vi "GetTaskTypeByTaskID.vi"(3 "Task ID":u32) -> (0 "task type":i32, 1 "Task ID":u32)   [LabVIEW 2009]
uses:
  Windows/System32/AdvLvDaq.dll
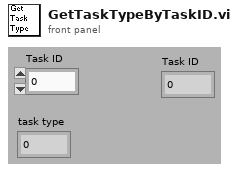
[diagram p1: front panel]
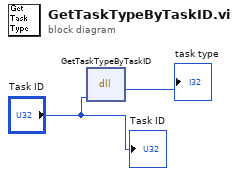
[diagram p0: block diagram]
diagram:
  n1 = dll-call lib="C:/Windows/System32/AdvLvDaq.dll" fn="GetTaskTypeByTaskID"("taskId"="Task ID") -> ("return type"=→"task type":i32)  [unwired: 4 in, 2 out]
  "Task ID" <- "Task ID"
